vi "joystick.vi"() -> ()   [LabVIEW 2017]
uses:
  <vilib>/myRIO/Common/Instrument Driver Framework/myRIO v1.0/UART/vis/myRIO v1.0 Close UART.vi
  <vilib>/Utility/inputDevices.llb/joystickAcquire.vi
  <vilib>/Utility/inputDevices.llb/closeJoystick.vi
  <vilib>/myRIO/Common/Instrument Driver Framework/Utilities/vis/FPGA Ref Manager.vi
  <vilib>/myRIO/Common/Instrument Driver Framework/myRIO v1.0/myRIO v1.0 Reset FPGA.vi
  <vilib>/myRIO/Common/Instrument Driver Framework/myRIO v1.0/IRQ/vis/myRIO v1.0 IRQ Info FGV.vi
  <vilib>/myRIO/Common/Instrument Driver Framework/myRIO v1.0/IRQ/vis/myRIO v1.0 Timer IRQ Info FGV.vi
  <vilib>/myRIO/Instrument Drivers/Utilities/Utilities.lvlib
panel:
  out "axis info":T1
  out "direction info":T2
  out "button info":T3
  in  "stop":bool
  # "Cross (-1 - none; 0 - up; 90 - right; 180 - down; 270 - left)"
  # "Button:"
  # "Left stick"
  # "1 - A"
  # "2 - B"
  # "Triggers"
  # "3 - X"
  # "Right stick"
  # "4 - Y"
  # "5 - LB"
  # "6 - RB"
  # "7 - SELECT"
  # "8 - START"
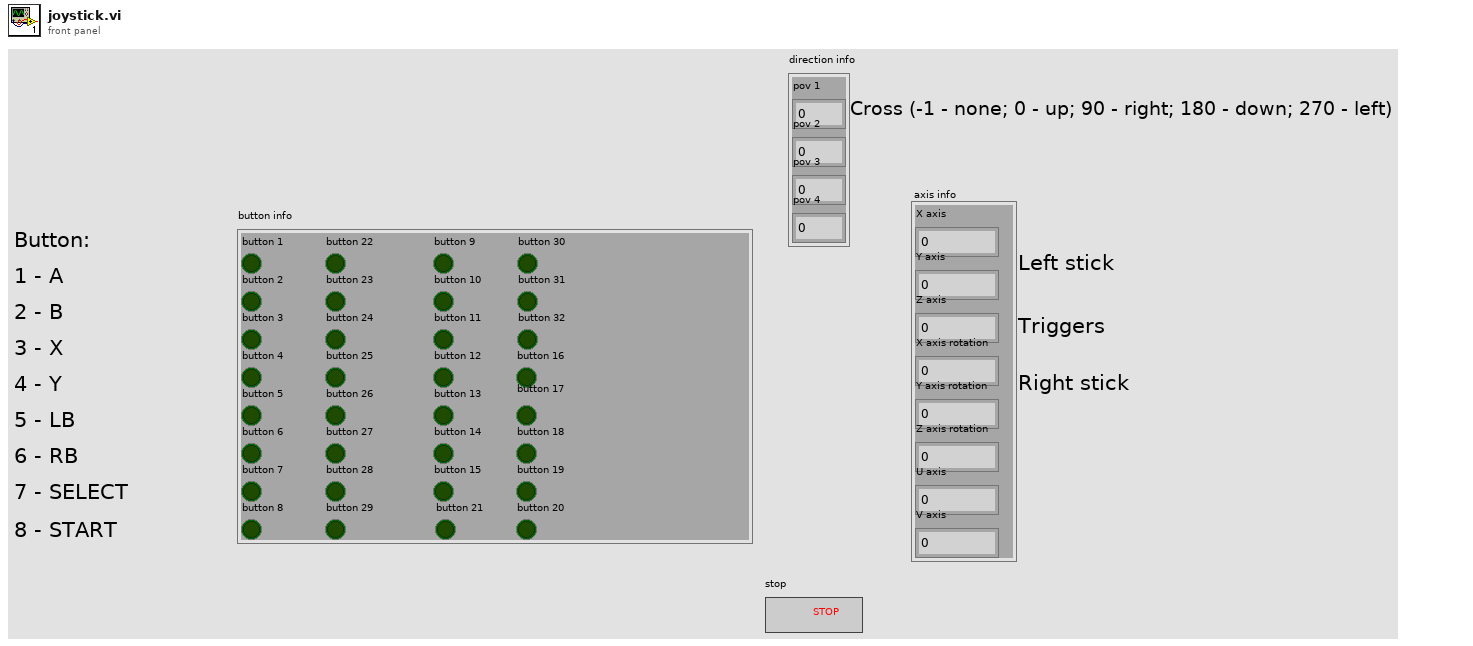
[diagram p1: front panel]
types:
  T1 = cluster{"X axis":i32, "Y axis":i32, "Z axis":i32, "X axis rotation":i32, "Y axis rotation":i32, "Z axis rotation":i32, "U axis":i32, "V axis":i32}
  T2 = cluster{"pov 1":i32, "pov 2":i32, "pov 3":i32, "pov 4":i32}
  T3 = cluster{"button 1":bool, "button 2":bool, "button 3":bool, "button 4":bool, "button 5":bool, "button 6":bool, "button 7":bool, "button 8":bool, "button 9":bool, "button 10":bool, "button 11":bool, "button 12":bool, "button 13":bool, "button 14":bool, "button 15":bool, "button 16":bool, "button 17":bool, "button 18":bool, "button 19":bool, "button 20":bool, "button 21":bool, "button 22":bool, "button 23":bool, "button 24":bool, "button 25":bool, "button 26":bool, "button 27":bool, "button 28":bool, "button 29":bool, "button 30":bool, "button 31":bool, "button 32":bool}
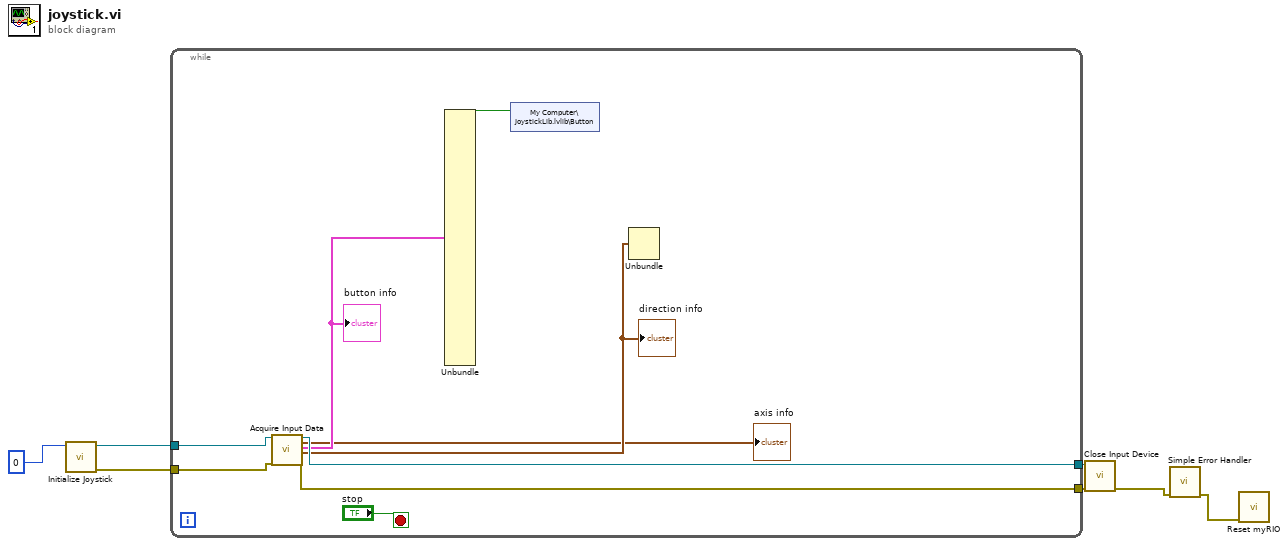
[diagram p0: block diagram]
diagram:
  n1 = call <vilib>:"Initialize Joystick.vi"("device index"=0) -> ("error out"=w3:errorcluster, "device ID"=w1:refnum<k1>)  [unwired: 9 in]
  n2 = while {
    tunnel: [w16] -> w7
    tunnel: [w15] -> w6
    tunnel: w3 -> [w14]
    tunnel: w1 -> [w12]
    stop <- "stop" stop-if-true
    n3 = call-poly <vilib>:"Acquire Input Data.vi"("device ID"=w12, "error in (no error)"=w14) -> ("device ID"=w16:refnum<k1>, "axis info"=→"axis info":T1, "button info"=w11:T3, "direction info"=w10:T2, "error out"=w15:errorcluster)  [unwired: 13 in]
    "button info" <- w11
    "direction info" <- w10
    n4 = Unbundle(w11) -> ("button 1"=w8:bool)  [unwired: 31 out]
    n5 = shared-variable "My Computer\\JoystickLib.lvlib\\Button"(w8) -> ()  [unwired: 1 in, 1 out]
    n6 = Unbundle(w10) -> ()  [unwired: 4 out]
  }
  n7 = call-poly <vilib>:"Close Input Device.vi"("error in (no error)"=w6, "device ID"=w7) -> ("error out"=w5:errorcluster)  [unwired: 8 in]
  n8 = call <vilib>:"Simple Error Handler.vi"("error in (no error)"=w5) -> ("error out"=w4:errorcluster)  [unwired: 4 in, 4 out]
  n9 = call <vilib>:"Reset myRIO.vi"("error in (no error)"=w4) -> ()  [unwired: 10 in, 1 out]
